vi "BRig_dataCurrent_Cue2Switch_LED.vi"() -> (2 "output_Cue2Switch_LED":i32)   [LabVIEW 2014]
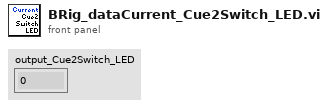
[diagram p1: front panel]
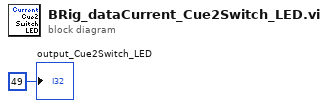
[diagram p0: block diagram]
diagram:
  "output_Cue2Switch_LED" <- 49 ("output_iBlock")
